vi "Initialize 1 Pin.vi"(8 "error in":errorcluster, 9 "Initialize_Info":T1, 10 "pin or relay name":string, 11 "measure call context in":refnum<class "Measure Call Context.lvclass">) -> (0 "error out":errorcluster, 1 "instrument objects":refnum<class "Abstract_Instrument.lvclass">[](array[class]), 2 "session reservation out":refnum<class "Session Reservation.lvclass">, 3 "measure call context out":refnum<class "Measure Call Context.lvclass">)   [LabVIEW 2021, in "Abstract_Instrument.lvclass"]
uses:
  Abstract_Instrument.lvclass
  controls/Initialize_Info.ctl
  <vilib>/Plug-In SDKs/Clients/Session Management V1/Session Reservation/Initialize and Close Session Behavior.ctl
  <vilib>/Plug-In SDKs/Measurements/Measure Call Context/Measure Call Context.lvclass
  <vilib>/Plug-In SDKs/Clients/Session Management V1/Session Reservation/Session Reservation.lvclass
  <vilib>/Plug-In SDKs/Measurements/Measure Call Context/Reserve Sessions - 1Pin.vi
  Reusables/Get Pin Information.lvlib
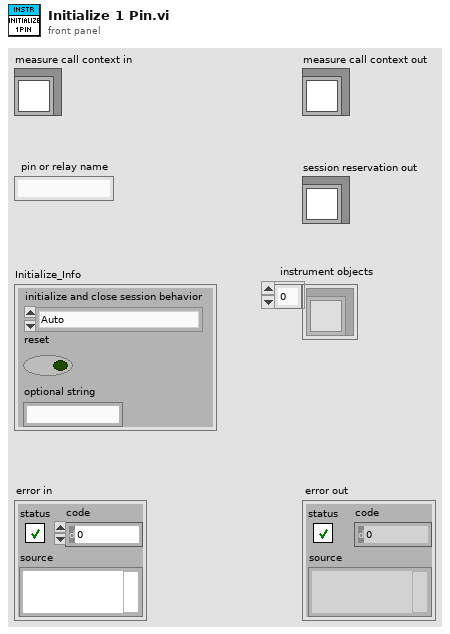
[diagram p1: front panel]
types:
  T1 = typedef "Abstract_Instrument.lvclass/Initialize_Info.ctl" = cluster{"initialize and close session behavior":T2, "reset":bool, "optional string":string}
  T2 = typedef "NI Session Management V1 Client.lvlib/Session Reservation.lvclass/Initialize and Close Session Behavior.ctl" = enum16{"Auto", "Initialize and Close", "Attach and Detach", "Initialize and Detach", "Attach and Close"}
  T3 = typedef "ni.measurementlink.sessionmanagement.v1.api.lvlib/ni_measurementlink_sessionmanagement_v1_ChannelMapping.ctl" = cluster{"pin_or_relay_name":string, "site":i32, "channel":string, "multiplexer_resource_name":string, "multiplexer_route":string}
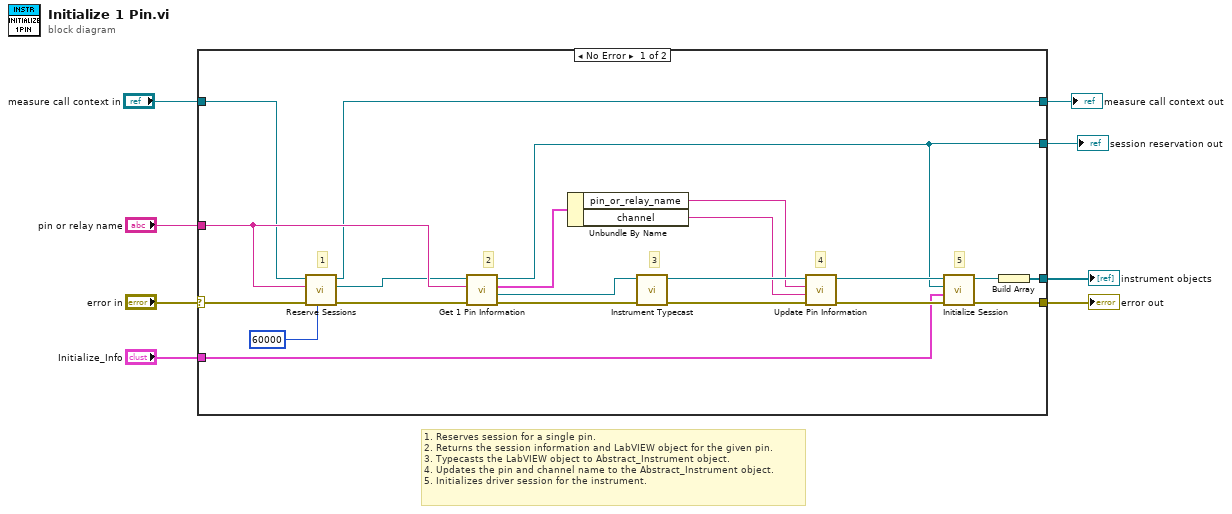
[diagram p0: block diagram]
diagram:
  # "1. Reserves session for a single pin.\n2. Returns the session information and LabVIEW object for the given pin.\n3. Typecasts the LabVIEW object to Abstract_Instrument object.\n4. Updates the pin and channel name to the Abstract_Instrument object.\n5. Initializes driver session for the instrument."
  n1 = case shown="No Error" "error in" {
    selector: "error in" -> [w17 w31]
    tunnel: [w21 _] -> w8
    tunnel: "Initialize_Info" -> [w20 _]
    tunnel: [w19 w31] -> w6
    tunnel: "pin or relay name" -> [w14 _]
    tunnel: [w12 _] -> w3
    tunnel: "measure call context in" -> [w11 w30]
    tunnel: [w10 w30] -> w1
    frame No Error {
      # "5"
      # "4"
      # "3"
      # "2"
      # "1"
      n2 = call-poly <vilib>:"Reserve Sessions.vi"("timeout (ms)"=60000, "error in"=w17, "pin or relay name"=w14, "measurement context in"=w11) -> ("error out"=w16:errorcluster, "session reservation out"=w9:refnum<class "Session Reservation.lvclass">, "measurement context out"=w10:refnum<class "Measure Call Context.lvclass">)  [unwired: 5 in]
      n3 = call "Get 1 Pin Information.vi"("error in"=w16, "pin or relay name"=w14, "session reservation in"=w9) -> ("error out"=w29:errorcluster, "pin instrument"=w18:refnum<class>, "channel_mappings"=w26:T3, "session reservation our"=w21:refnum<class "Session Reservation.lvclass">)  [unwired: 5 in]
      n4 = Unbundle By Name(w26) -> ("pin_or_relay_name"=w25:string, "channel"=w24:string)
      n5 = call "Instrument Typecast.vi"("error in (no error)"=w29, "pin instrument"=w18) -> ("error out"=w28:errorcluster, "instrument object"=w27:refnum<class "Abstract_Instrument.lvclass">)  [unwired: 8 in]
      n6 = call "Update Pin Information.vi"("error in"=w28, "channel"=w24, "pin_name"=w25, "instrument object in"=w27) -> ("error out"=w23:errorcluster, "instrument object out"=w22:refnum<class "Abstract_Instrument.lvclass">)  [unwired: 6 in]
      n7 = call-dynamic "Initialize Session.vi"("error in (no error)"=w23, "Initialize_Info"=w20, "session reservation in"=w21, "Abstract_Instrument in"=w22) -> ("error out"=w19:errorcluster, "Abstract_Instrument out"=w13:refnum<class "Abstract_Instrument.lvclass">)  [unwired: 6 in]
      n8 = Build Array(w13) -> (w12:refnum<class "Abstract_Instrument.lvclass">[])
    }
    frame Error {
    }
  }
  "error out" <- w6
  "instrument objects" <- w3
  "measure call context out" <- w1
  "session reservation out" <- w8
